vi "LattePanda Controller.vi"(8 "error in":errorcluster) -> ()   [LabVIEW 2018]
doc: "This VI executes continuously carrying out the current operation and responding to updates or new operations. It will often contain the timing or control code that is difficult to place directly in TeleOp. This VI generally opens all sensors and motors and isolates the rest of the robot code from knowing how the operations are carried out."
uses:
  <vilib>/Rock Robotics/WPI/Framework/Completion Status.ctl
  LattePanda Setpoints.ctl
  LattePanda Operations.ctl
  <vilib>/Rock Robotics/SystemInterfaces/DIO/FPGA_DIOChannel.ctl
  Commands/PowerOnStateMachineStates.ctl
  LattePanda Published Globals.vi
  <vilib>/Rock Robotics/Network Tables/NT Write Boolean.vi
panel:
  out "Waiting for Connection":bool
  out "Power Enabled?":bool
  out "NT Connection":bool
  out "Pingable":bool
  in  "Interactive Values":T1
  out "Current\nCmd":string
  in  "Buttons":cluster{"Execute Cmd":bool, "Abort Cmd":bool}
  out "Command Timing":cluster{"Start Time (ms)":u32, "Iterations":i32}
  out "Status":T3
  # "Tip: It may be helpful to observe inputs and sensor values.\nYou may also want to display tuning or debugging controls."
  # "Interactive Command: You may fill in the settings for a command\nand schedule it with the Execute button. You can observe and abort\nany command while fine tuning the code for the controller."
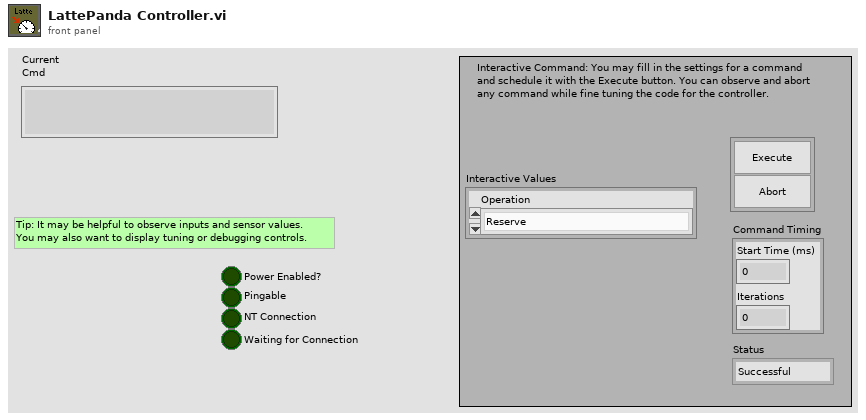
[diagram p1: front panel]
types:
  T1 = typedef "LattePanda Setpoints.ctl" = cluster{"Operation":T2}
  T2 = typedef "LattePanda Operations.ctl" = enum16{"Reserve", "Read Current", "Power On", "Shut Down", "Force Power Cycle", "Restart"}
  T3 = typedef "Completion Status.ctl" = enum16{"Successful", "Aborted", "Incomplete"}
  T4 = typedef "FPGA_DIOChannel.ctl" = enum8{"DIO 0", "DIO 1", "DIO 2", "DIO 3", "DIO 4", "DIO 5", "DIO 6", "DIO 7", "DIO 8", "DIO 9", "DIO MXP 0", "DIO MXP 1", "DIO MXP 2", "DIO MXP 3", "DIO MXP 4", "DIO MXP 5", "DIO MXP 6", "DIO MXP 7", "DIO MXP 8", "DIO MXP 9", "DIO MXP 10", "DIO MXP 11", "DIO MXP 12", "DIO MXP 13", "DIO MXP 14", "DIO MXP 15", "SPI Port CS1", "SPI Port CS2", "SPI Port CS3", "SPI Port MISO", "SPI Port MOSI", "Invalid"}
  T5 = typedef "WPI_DigitalOutputDevRef.ctl" = cluster{"DIO Channel":T4, "DevStatus":errorcluster}
  T6 = typedef "Command Status Info.ctl" = cluster{"Name":string, "Status":T3, "notifier out":T7}
  T7 = typedef "Completion Notifier.ctl" = refnum<notifier>
  T8 = cluster{"Current Command":T1, "Command Timing":cluster{"Start Time (ms)":u32, "Iterations":i32}, "Command Arguments":cluster{"Command Info":T6, "Description":string, "Default Command":T1, "queue out":refnum<queue>, "Subsystem Name":string}}
  T9 = typedef "PowerOnStateMachineStates.ctl" = enum16{"Idle", "Cycle Off", "Wait", "Cycle On", "Wait for Ping", "Wait for Power Off", "Power off grace period"}
  T10 = enum16{"Add Cnx", "Remove Cnx", "Retrieve List", "Cnx Inited"}
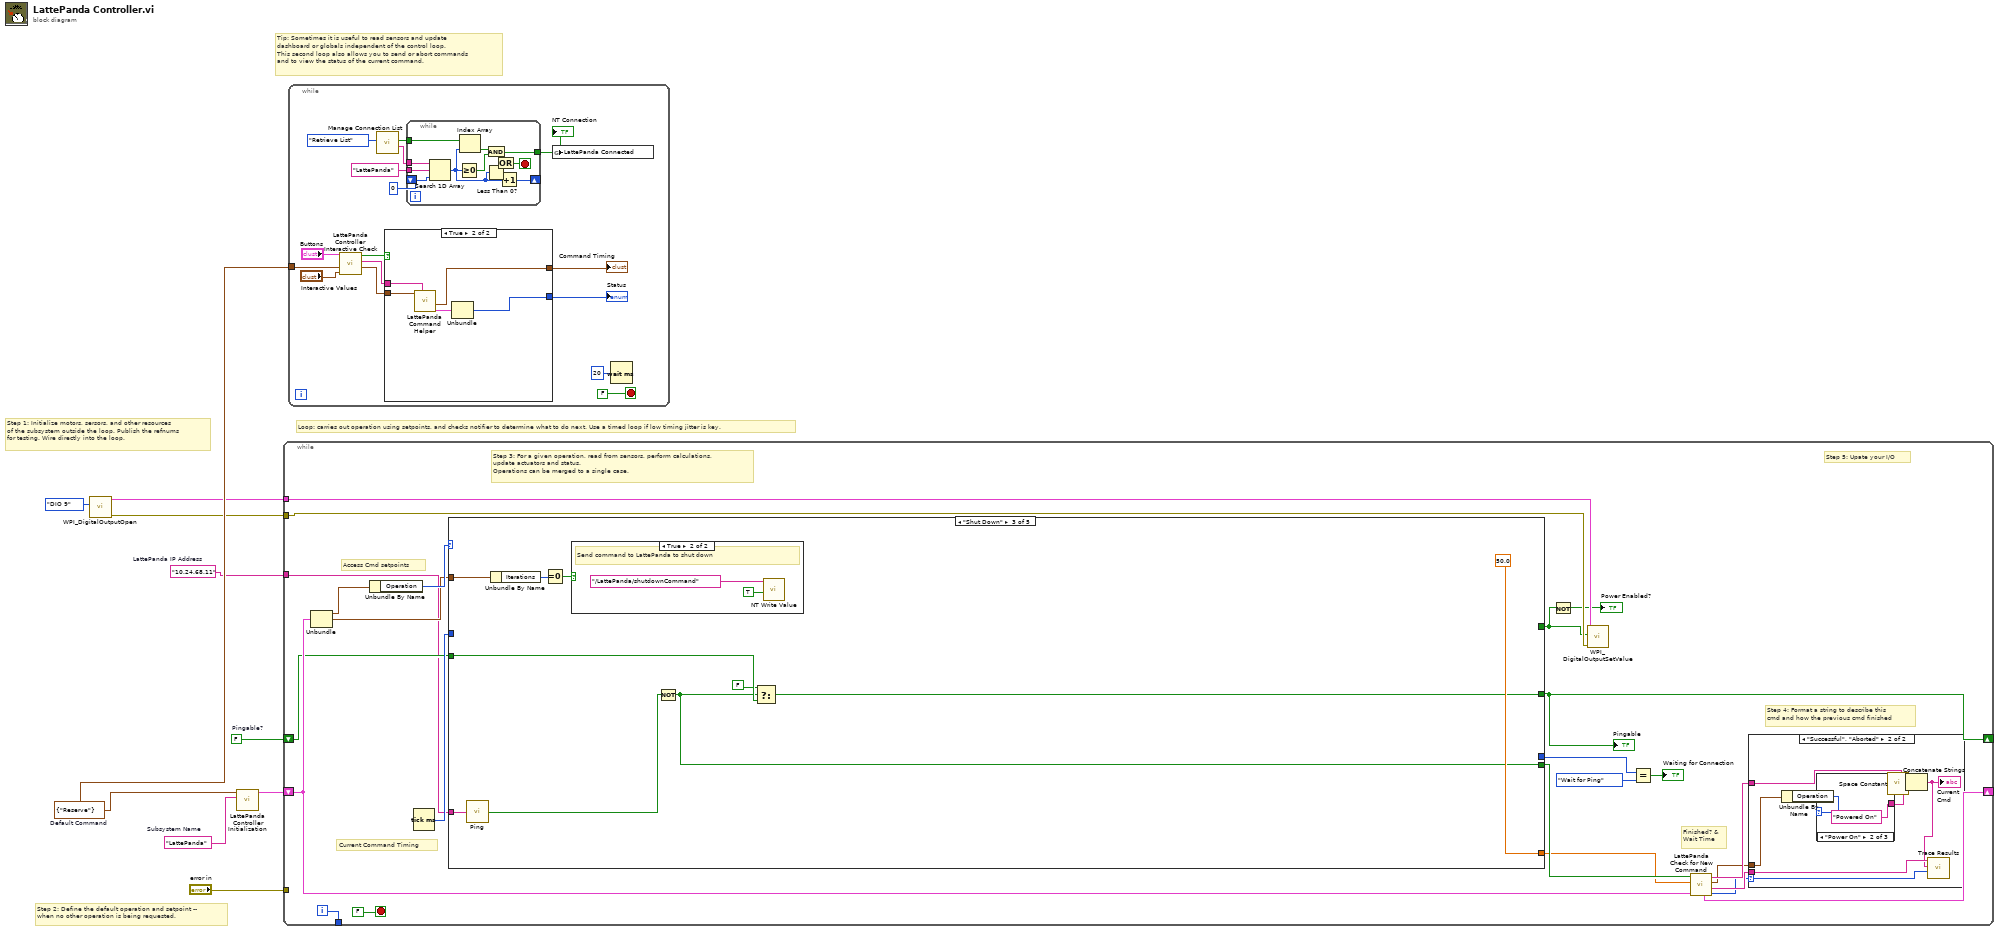
[diagram p0: block diagram]
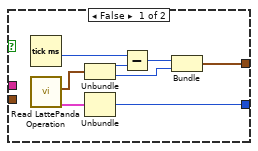
[diagram p2: hidden frame]
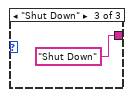
[diagram p5: hidden frame]
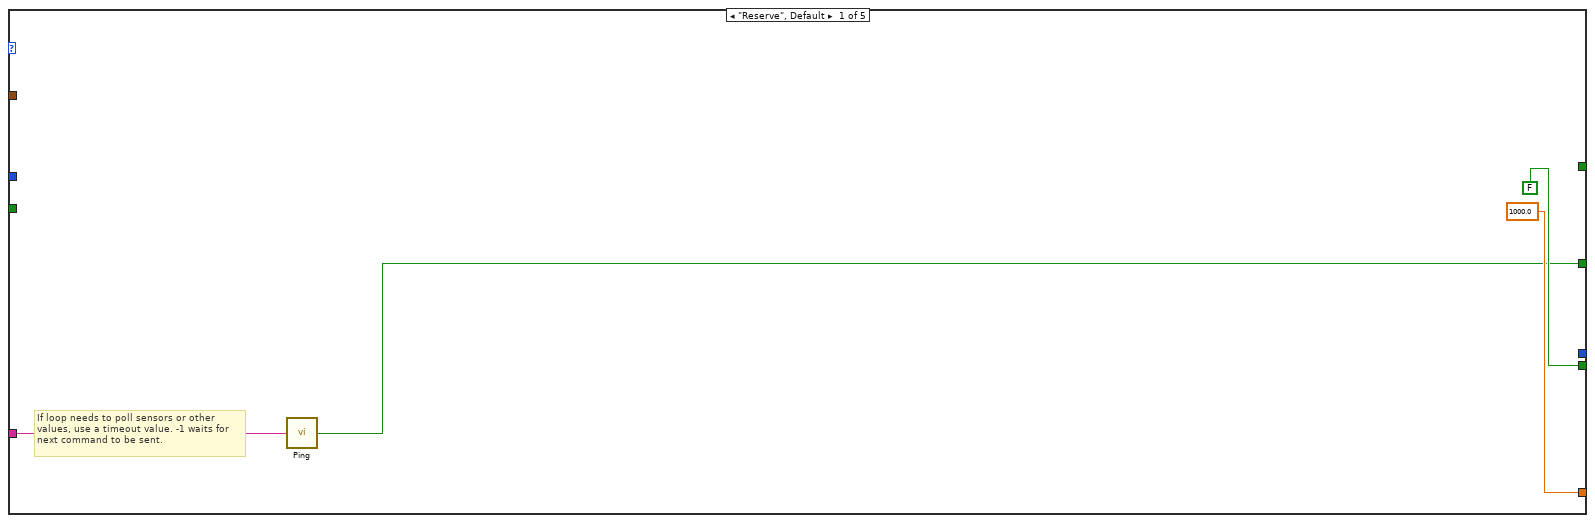
[diagram p6: hidden frame]
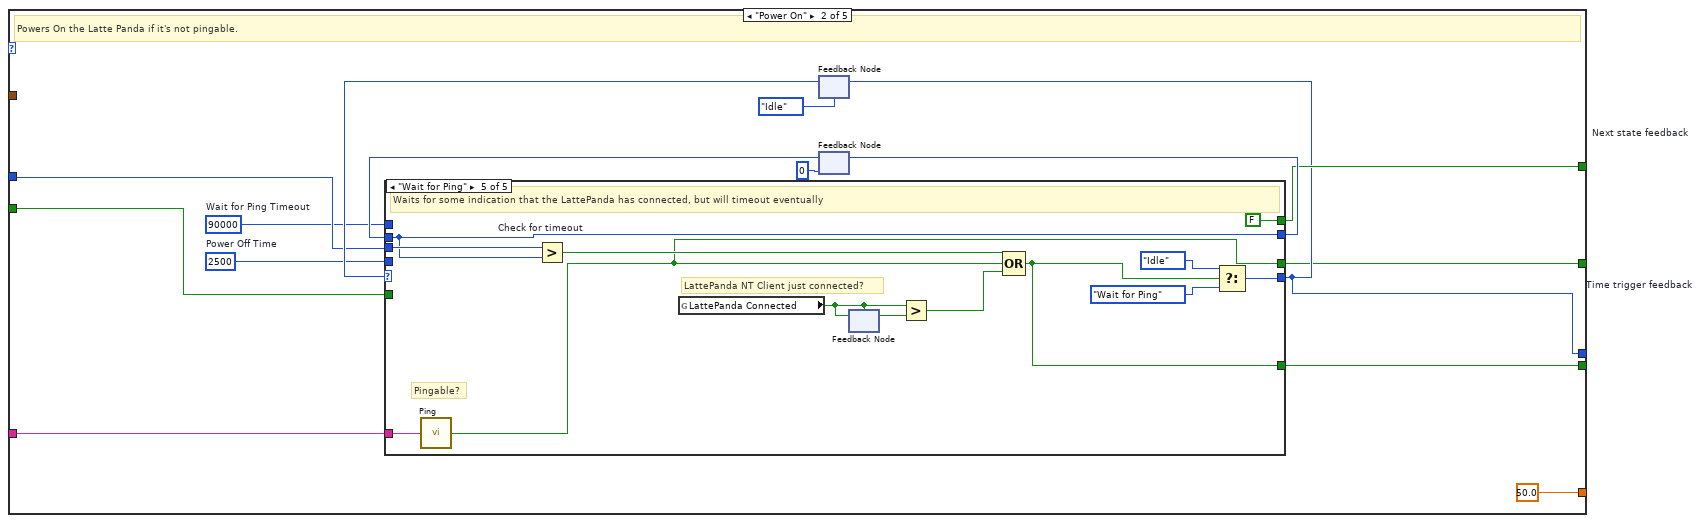
[diagram p7: hidden frame]
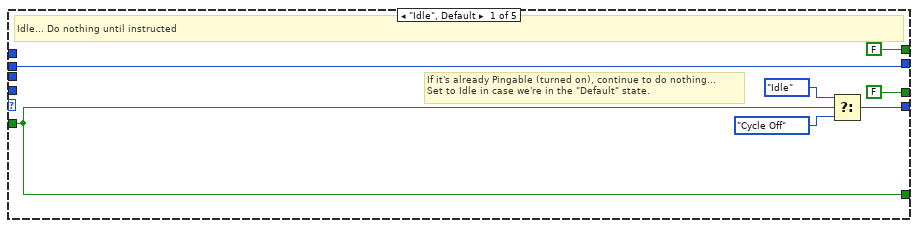
[diagram p8: hidden frame]
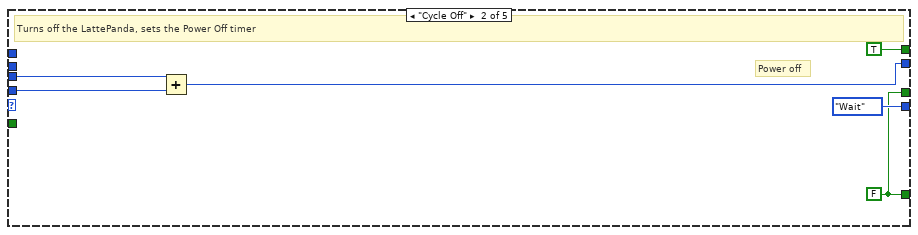
[diagram p9: hidden frame]
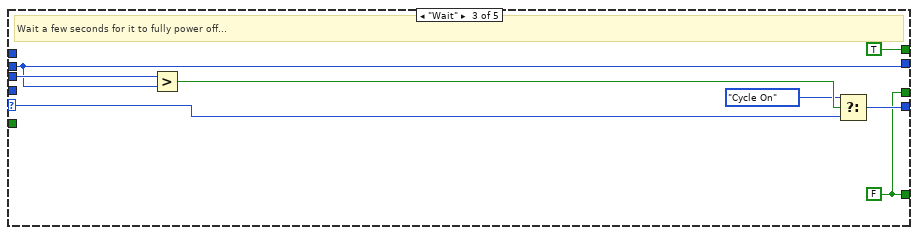
[diagram p10: hidden frame]
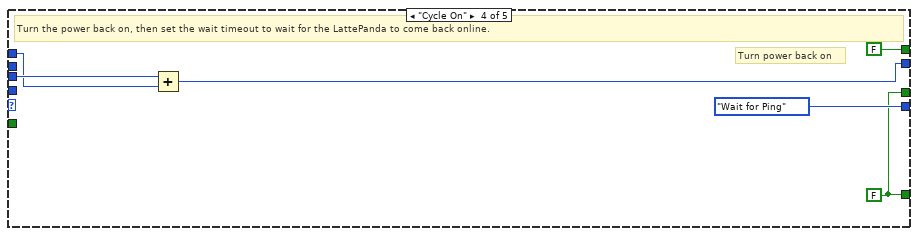
[diagram p11: hidden frame]
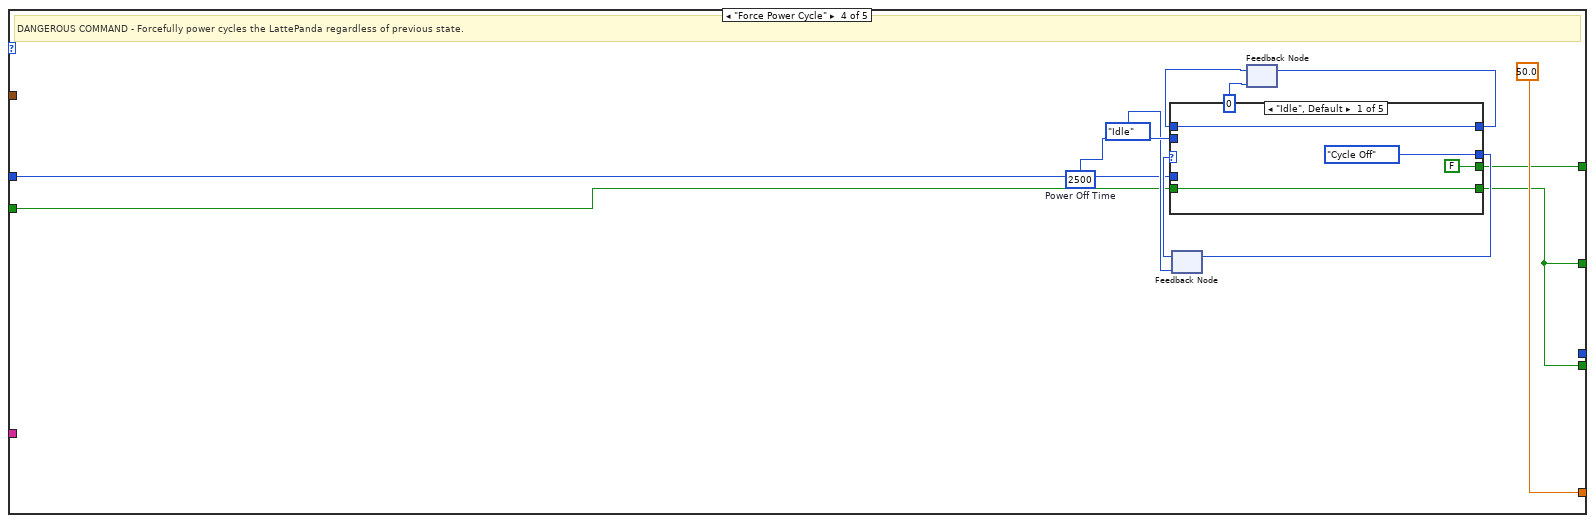
[diagram p13: hidden frame]
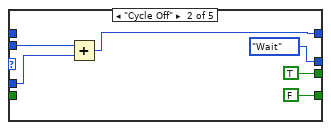
[diagram p14: hidden frame]
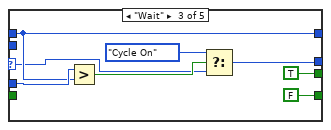
[diagram p15: hidden frame]
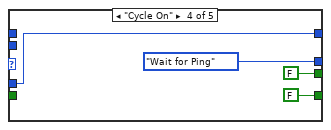
[diagram p16: hidden frame]
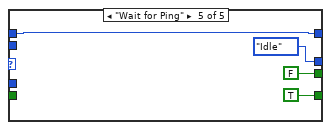
[diagram p17: hidden frame]
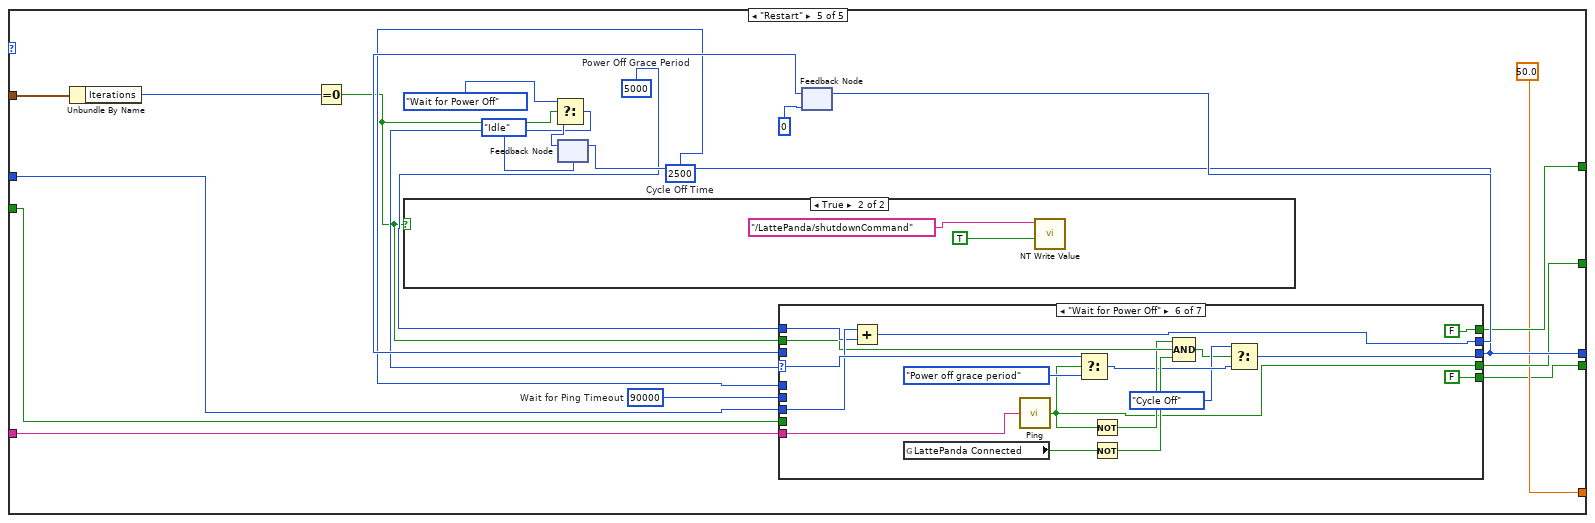
[diagram p18: hidden frame]
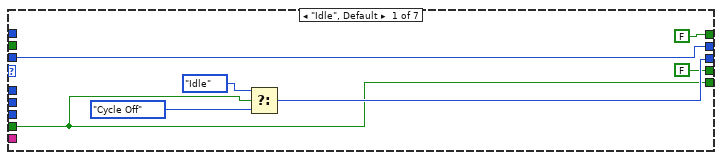
[diagram p19: hidden frame]
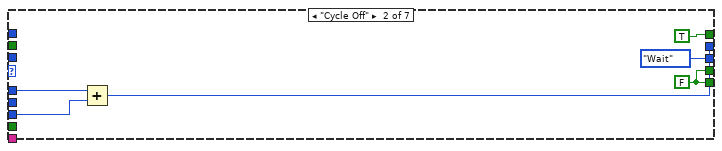
[diagram p20: hidden frame]
diagram:
  w1 = "10.24.68.11"  # LattePanda IP Address
  w2 = FALSE  # Pingable?
  w6 = T1 {"Operation"=enum."Reserve"}  # Default Command
  w7 = "LattePanda"  # Subsystem Name
  # "Tip: Sometimes it is useful to read sensors and update\ndashboard or globals independent of the control loop.\nThis second loop also allows you to send or abort commands\nand to view the status of the current command."
  # "Step 2: Define the default operation and setpoint --\nwhen no other operation is being requested."
  # "Step 1: Initialize motors, sersors, and other resources\nof the subsystem outside the loop. Publish the refnums\nfor testing. Wire directly into the loop."
  # "Loop: carries out operation using setpoints, and checks notifier to determine what to do next. Use a timed loop if low timing jitter is key."
  n1 = call <vilib>:"WPI_DigitalOutputOpen.vi"("DIO Channel"=FPGA_DIOChannel."DIO 9") -> ("error out"=w3:errorcluster, "DigitalOutputDevRef"=w4:T5)  [unwired: 9 in]
  n2 = call "LattePanda Controller Initialization.vi"("Subsystem Name"=w7, "Default Command"=w6) -> ("Current Command"=w8:T8)  [unwired: 9 in]
  n3 = while {
    shift-right: [w27] -> _
    shift-left: w8 -> [w20]
    tunnel: [w32] -> _
    tunnel: "error in" -> [_]
    tunnel: w4 -> [w16]
    tunnel: w3 -> [w15]
    shift-right: [w18] -> _
    shift-left: w2 -> [w19]
    tunnel: w1 -> [w17]
    i -> [w32]
    stop <- FALSE stop-if-true
    # "Step 5: Upate your I/O"
    # "Step 4: Format a string to describe this\ncmd and how the previous cmd finished"
    # "Current Command Timing"
    # "Access Cmd setpoints"
    # "Finished? &\nWait Time"
    # "Step 3: For a given operation, read from sensors, perform calculations,\nupdate actuators and status.\nOperations can be merged to a single case."
    n4 = Unbundle(w20) -> ("Current Command"=w31:T1, "Command Timing"=w28:cluster{"Start Time (ms)":u32, "Iterations":i32})  [unwired: 1 out]
    n5 = Unbundle By Name(w31) -> ("Operation"=w30:T2)
    n6 = Tick Count (ms)() -> (millisecond timer value=w29:u32)
    n7 = case shown="\"Shut Down\"" w30 {
      tunnel: [1000.0 ("Infinite") 50.0 ("Infinite") 50.0 ("Infinite") 50.0 ("Infinite") 50.0 ("Infinite")] -> w25
      tunnel: [FALSE ("ignore previous (F)") w53 w103 w115 w153] -> w26
      tunnel: w28 -> [_ _ w112 _ w172]
      tunnel: w29 -> [_ w59 _ w119 w157]
      tunnel: w19 -> [_ w60 w108 w118 w156]
      tunnel: [w45 w48 w106 w115 w163] -> w18
      tunnel: w17 -> [w44 w52 w105 _ w158]
      tunnel: [_ w54 _ w116 w165] -> w14
      tunnel: [_ w49 _ _ w164] -> w13
      frame "Reserve", Default {
        # "If loop needs to poll sensors or other\nvalues, use a timeout value. -1 waits for\nnext command to be sent."
        n8 = call "Ping.vi"("IP Address"=w44) -> ("Found?"=w45:bool)
      }
      frame "Power On" {
        w50 = u32 2500  # Power Off Time
        w51 = u32 90000  # Wait for Ping Timeout
        # "Powers On the Latte Panda if it's not pingable."
        n9 = feedback #1 "Next state feedback"(PowerOnStateMachineStates."Idle") -> (w61:T9)
        n10 = feedback #2 "Time trigger feedback"(u32 0) -> (w57:u32)
        n11 = case shown="\"Wait for Ping\"" w61 {
          selector: w61 -> [_ _ w77 _ _]
          tunnel: w60 -> [w64 _ _ _ _]
          tunnel: [w69 PowerOnStateMachineStates."Wait" w81 PowerOnStateMachineStates."Wait for Ping" w99] -> w49
          tunnel: w59 -> [_ w71 w83 w87 w102]
          tunnel: [w65 w75 w79 w86 w96] -> w58
          tunnel: w57 -> [w65 _ w79 _ w96]
          tunnel: [FALSE ("Value") TRUE ("Value") TRUE ("Value") FALSE FALSE ("Value")] -> w54
          tunnel: [w64 w72 w76 w84 w94] -> w53
          tunnel: w52 -> [_ _ _ _ w97]
          tunnel: w51 -> [_ _ _ w85 _]
          tunnel: w50 -> [_ w70 _ _ _]
          tunnel: [FALSE ("Found?") w72 w76 w84 w90] -> w48
          frame "Idle", Default {
            # "If it's already Pingable (turned on), continue to do nothing...\nSet to Idle in case we're in the \"Default\" state."
            # "Idle... Do nothing until instructed"
            n12 = Select(t=PowerOnStateMachineStates."Idle", s=w64, f=PowerOnStateMachineStates."Cycle Off") -> (s? t:f=w69:T9)
          }
          frame "Cycle Off" {
            w72 = FALSE
            # "Power off"
            # "Turns off the LattePanda, sets the Power Off timer"
            n13 = Add(x=w71, y=w70) -> (x+y=w75:u32)
          }
          frame "Wait" {
            w76 = FALSE
            # "Wait a few seconds for it to fully power off..."
            n14 = Greater?(x=w83, y=w79) -> (0:w82:bool)
            n15 = Select(t=PowerOnStateMachineStates."Cycle On", s=w82, f=w77) -> (s? t:f=w81:T9)
          }
          frame "Cycle On" {
            w84 = FALSE
            # "Turn power back on"
            # "Turn the power back on, then set the wait timeout to wait for the LattePanda to come back online."
            n16 = Add(x=w87, y=w85) -> (x+y=w86:u32)
          }
          frame "Wait for Ping" {
            # "Pingable?"
            # "LattePanda NT Client just connected?"
            # "Waits for some indication that the LattePanda has connected, but will timeout eventually"
            n17 = call "Ping.vi"("IP Address"=w97) -> ("Found?"=w90:bool)
            n18 = Greater? "Check for timeout"(x=w102, y=w96) -> (0:w93:bool)
            n19 = global read "LattePanda Published Globals.vi" "LattePanda Connected"() -> (w91:bool)
            n20 = feedback-in #3(w91) -> ()
            n21 = feedback #3(w91) -> (w95:bool)
            n22 = Greater?(x=w91, y=w95) -> (0:w92:bool)
            n23 = Compound Arithmetic op=OR(w93, w90, w92) -> (w94:bool)
            n24 = Select(t=PowerOnStateMachineStates."Idle", s=w94, f=PowerOnStateMachineStates."Wait for Ping") -> (s? t:f=w99:T9)
          }
        }
        n25 = feedback-in #1(w49) -> ()
        n26 = feedback-in #2(w58) -> ()
      }
      frame "Shut Down" {
        n27 = call "Ping.vi"("IP Address"=w105) -> ("Found?"=w104:bool)
        n28 = Unbundle By Name(w112) -> ("Iterations"=w110:i32)
        n29 = Equal To 0?(x=w110) -> (x = 0?=w111:bool)
        n30 = case shown="True" w111 {
          frame False {
          }
          frame True {
            # "Send command to LattePanda to shut down"
            n31 = call-poly <vilib>:"NT Write Value.vi"("Boolean"=TRUE, "Name"="/LattePanda/shutdownCommand") -> ()  [unwired: 9 in, 1 out]
          }
        }
        n32 = Not(x=w104) -> (.not. x?=w103:bool)
        n33 = Select(t=FALSE, s=w103, f=w108) -> (s? t:f=w106:bool)
      }
      frame "Force Power Cycle" {
        w124 = u32 2500  # Power Off Time
        # "DANGEROUS COMMAND - Forcefully power cycles the LattePanda regardless of previous state."
        n34 = feedback #4(PowerOnStateMachineStates."Idle") -> (w125:T9)
        n35 = feedback #5(u32 0) -> (w126:u32)
        n36 = case shown="\"Idle\", Default" w125 {
          selector: w125 -> [_ _ w137 _ _]
          tunnel: w118 -> [w128 _ _ _ _]
          tunnel: [PowerOnStateMachineStates."Cycle Off" PowerOnStateMachineStates."Wait" w142 PowerOnStateMachineStates."Wait for Ping" PowerOnStateMachineStates."Idle"] -> w121
          tunnel: w119 -> [_ w136 w144 w145 _]
          tunnel: [w129 w135 w140 w145 w151] -> w120
          tunnel: w126 -> [w129 _ w140 _ w151]
          tunnel: [w128 FALSE FALSE FALSE TRUE] -> w115
          tunnel: w124 -> [_ w131 _ _ _]
          tunnel: [FALSE ("Value") TRUE ("Value") TRUE ("Value") FALSE FALSE ("Value")] -> w116
          frame "Idle", Default {
          }
          frame "Cycle Off" {
            n37 = Add(x=w131, y=w136) -> (x+y=w135:u32)
          }
          frame "Wait" {
            n38 = Greater?(x=w144, y=w140) -> (0:w143:bool)
            n39 = Select(t=PowerOnStateMachineStates."Cycle On", s=w143, f=w137) -> (s? t:f=w142:T9)
          }
          frame "Cycle On" {
          }
          frame "Wait for Ping" {
          }
        }
        n40 = feedback-in #4(w121) -> ()
        n41 = feedback-in #5(w120) -> ()
      }
      frame "Restart" {
        w155 = u32 5000  # Power Off Grace Period
        w166 = u32 2500  # Cycle Off Time
        w167 = u32 90000  # Wait for Ping Timeout
        n42 = Unbundle By Name(w172) -> ("Iterations"=w173:i32)
        n43 = Equal To 0?(x=w173) -> (x = 0?=w154:bool)
        n44 = case shown="True" w154 {
          frame False {
          }
          frame True {
            n45 = call-poly <vilib>:"NT Write Value.vi"("Boolean"=TRUE, "Name"="/LattePanda/shutdownCommand") -> ()  [unwired: 9 in, 1 out]
          }
        }
        n46 = feedback #6(PowerOnStateMachineStates."Idle") -> (w161:T9)
        n47 = Select(t=PowerOnStateMachineStates."Wait for Power Off", s=w154, f=w161) -> (s? t:f=w159:T9)
        n48 = feedback #7(u32 0) -> (w169:u32)
        n49 = case shown="\"Wait for Power Off\"" w159 {
          selector: w159 -> [_ _ w188 _ _ w229 w235]
          tunnel: w156 -> [w175 _ _ _ _ _ _]
          tunnel: [w180 PowerOnStateMachineStates."Wait" w192 PowerOnStateMachineStates."Wait for Ping" w210 w216 w237] -> w164
          tunnel: w157 -> [_ w186 w194 w198 w213 w226 w239]
          tunnel: [w176 w185 w190 w197 w207 w224 w233] -> w170
          tunnel: w169 -> [w176 _ w190 _ w207 _ w233]
          tunnel: [FALSE ("Value") TRUE ("Value") TRUE ("Value") FALSE FALSE ("Value") FALSE ("Value") FALSE ("Value")] -> w165
          tunnel: [w175 w181 w187 w195 w205 FALSE ("Pingable?") FALSE ("Pingable?")] -> w153
          tunnel: w158 -> [_ _ _ _ w208 w230 _]
          tunnel: w167 -> [_ _ _ w196 _ _ _]
          tunnel: w166 -> [_ w182 _ _ _ _ _]
          tunnel: [FALSE ("Found?") w181 w187 w195 w201 w218 FALSE ("Found?")] -> w163
          tunnel: w155 -> [_ _ _ _ _ w225 _]
          tunnel: w154 -> [_ _ _ _ _ w222 _]
          frame "Idle", Default {
            n50 = Select(t=PowerOnStateMachineStates."Idle", s=w175, f=PowerOnStateMachineStates."Cycle Off") -> (s? t:f=w180:T9)
          }
          frame "Cycle Off" {
            w181 = FALSE
            n51 = Add(x=w182, y=w186) -> (x+y=w185:u32)
          }
          frame "Wait" {
            w187 = FALSE
            n52 = Greater?(x=w194, y=w190) -> (0:w193:bool)
            n53 = Select(t=PowerOnStateMachineStates."Cycle On", s=w193, f=w188) -> (s? t:f=w192:T9)
          }
          frame "Cycle On" {
            w195 = FALSE
            n54 = Add(x=w198, y=w196) -> (x+y=w197:u32)
          }
          frame "Wait for Ping" {
            n55 = Greater?(x=w213, y=w207) -> (0:w204:bool)
            n56 = call "Ping.vi"("IP Address"=w208) -> ("Found?"=w201:bool)
            n57 = global read "LattePanda Published Globals.vi" "LattePanda Connected"() -> (w202:bool)
            n58 = feedback-in #8(w202) -> ()
            n59 = feedback #8(w202) -> (w206:bool)
            n60 = Greater?(x=w202, y=w206) -> (0:w203:bool)
            n61 = Compound Arithmetic op=OR(w204, w201, w203) -> (w205:bool)
            n62 = Select(t=PowerOnStateMachineStates."Idle", s=w205, f=PowerOnStateMachineStates."Wait for Ping") -> (s? t:f=w210:T9)
          }
          frame "Wait for Power Off" {
            n63 = Add(x=w226, y=w225) -> (x+y=w224:u32)
            n64 = global read "LattePanda Published Globals.vi" "LattePanda Connected"() -> (w220:bool)
            n65 = call "Ping.vi"("IP Address"=w230) -> ("Found?"=w218:bool)
            n66 = Select(t=w229, s=w218, f=PowerOnStateMachineStates."Power off grace period") -> (s? t:f=w217:T9)
            n67 = Not(x=w218) -> (.not. x?=w221:bool)
            n68 = Not(x=w220) -> (.not. x?=w219:bool)
            n69 = Compound Arithmetic op=AND(w221, w222, w219) -> (w214:bool)
            n70 = Select(t=PowerOnStateMachineStates."Cycle Off", s=w214, f=w217) -> (s? t:f=w216:T9)
          }
          frame "Power off grace period" {
            n71 = Greater?(x=w239, y=w233) -> (0:w238:bool)
            n72 = Select(t=PowerOnStateMachineStates."Cycle Off", s=w238, f=w235) -> (s? t:f=w237:T9)
          }
        }
        n73 = feedback-in #6(w164) -> ()
        n74 = feedback-in #7(w170) -> ()
      }
    }
    "Pingable" <- w18
    n75 = Not(x=w14) -> (.not. x?=→"Power Enabled?":bool)
    n76 = call <vilib>:"WPI_DigitalOutputSetValue.vi"("error in (no error)"=w15, "Value"=w14, "DigitalOutputDevRef"=w16) -> ()  [unwired: 7 in, 2 out]
    n77 = Equal?(x=w13, y=PowerOnStateMachineStates."Wait for Ping") -> (x = y?=→"Waiting for Connection":bool)
    n78 = call "LattePanda Check for New Command.vi"("Current Command"=w20, "Wait time (ms)"=w25, "Finished?"=w26) -> ("Completion"=w21:T3, "Subsystem Name"=w22:string, "Current Command"=w23:T1, "Initial Trace String"=w24:string, "NextCommand"=w27:T8)  [unwired: 4 in]
    n79 = case shown="\"Successful\", \"Aborted\"" w21 {
      selector: w21 -> [_ w41]
      tunnel: w24 -> [_ w37]
      tunnel: w23 -> [_ w40]
      tunnel: w22 -> [_ w39]
      frame "Incomplete", Default {
        # "Continuing current command"
      }
      frame "Successful", "Aborted" {
        # "Report and setup for next command"
        n80 = Unbundle By Name(w40) -> ("Operation"=w38:T2)
        n81 = case shown="\"Power On\"" w38 {
          tunnel: [_ "Powered On" "Shut Down"] -> w35
          frame "Reserve", Default {
          }
          frame "Power On" {
          }
          frame "Shut Down" {
          }
        }
        n82 = call <vilib>:"Space Constant.vi"() -> ("String"=w36:string)
        n83 = Concatenate Strings(w37, w36, w35) -> (w34:string)
        "Current\nCmd" <- w34
        n84 = call <vilib>:"Trace Results.vi"("Status of previous command"=w41, "Description"=w34, "Subsystem"=w39) -> ()  [unwired: 9 in]
      }
    }
  }
  n85 = while {
    tunnel: w6 -> [w254]
    stop <- FALSE stop-if-true
    n86 = call "LattePanda Controller Interactive Check.vi"("Interactive Command in"="Interactive Values", "Default Command"=w254, "Buttons"="Buttons") -> ("Interactive Command out"=w251:T1, "Trace String"=w252:string, "Schedule"=w253:bool)  [unwired: 6 in]
    n87 = call <vilib>:"Manage Connection List.vi"("Operation"=T10."Retrieve List") -> ("Names"=w246:string[], "Inited"=w244:bool[])  [unwired: 8 in, 1 out]
    n88 = case shown="True" w253 {
      tunnel: [w276 w281] -> w250
      tunnel: w251 -> [_ w279]
      tunnel: [w269 w277] -> w249
      tunnel: w252 -> [_ w280]
      frame False {
        n89 = Tick Count (ms)() -> (millisecond timer value=w272:u32)
        n90 = call "Read LattePanda Operation.vi"() -> ("Command Info"=w271:T6, "Command Timing"=w270:cluster{"Start Time (ms)":u32, "Iterations":i32})  [unwired: 9 in, 1 out]
        n91 = Unbundle(w270) -> ("Start Time (ms)"=w275:u32, "Iterations"=w273:i32)
        n92 = Unbundle(w271) -> ("Status"=w276:T3)  [unwired: 2 out]
        n93 = Subtract(x=w272, y=w275) -> (x-y=w274:u32)
        n94 = Bundle(w274, "Iterations"=w273) -> (w269:cluster{u32, "Iterations":i32})  [unwired: 1 in]
      }
      frame True {
        n95 = call "LattePanda Command Helper.vi"("Description"=w280, "SubSystem Data"=w279) -> ("Command Info Out"=w278:T6, "Command Timing"=w277:cluster{"Start Time (ms)":u32, "Iterations":i32})  [unwired: 7 in, 1 out]
        n96 = Unbundle(w278) -> ("Status"=w281:T3)  [unwired: 2 out]
      }
    }
    "Status" <- w250
    "Command Timing" <- w249
    n97 = while {
      tunnel: w246 -> [w268]
      tunnel: "LattePanda" ("element") -> [w267]
      tunnel: w244 -> [w266]
      tunnel: [w261] -> w243
      shift-right: [w258] -> _
      shift-left: 0 -> [w263]
      stop <- w262 stop-if-true
      n98 = Search 1D Array(1D array=w268, element=w267, start index (0)=w263) -> (index of element=w260:i32)
      n99 = Greater Or Equal To 0?(x=w260) -> (x >= 0?=w264:bool)
      n100 = Index Array(array=w266, index=w260) -> (element=w265:bool)
      n101 = And(x=w265, y=w264) -> (x .and. y?=w261:bool)
      n102 = Less Than 0?(x=w260) -> (x < 0?=w259:bool)
      n103 = Or(x=w261, y=w259) -> (x .or. y?=w262:bool)
      n104 = Increment(x=w260) -> (x+1=w258:i32)
    }
    "NT Connection" <- w243
    n105 = global write "LattePanda Published Globals.vi" "LattePanda Connected"(w243) -> ()
    n106 = Wait (ms)(milliseconds to wait=u32 20) -> ()  [unwired: 1 out]
  }
